vi "Dispense Function (SubVI).vi"(0 "Signals IN":T3={"Dispense"=FALSE, "Fill"=FALSE, "Spray"=FALSE, "Drain"=TRUE, "Complete"=FALSE, "Fill Error"=FALSE, "Dispense Error"=FALSE, "Fill Timeout"=FALSE, "Dispense Timeout"=FALSE}, 1 "Values IN":T4 {"Drain Time (s)" format="%.2f"; "Drain Rate (g/sec)" format="%.2f"; "Time Elapsed (s)" format="%.2f"; "Time Target (s)" format="%.2f"; "Dynamic Setpoint (g)" format="%.2f"; "Static Setpoint (g)" format="%.2f"; "Grams to Setpoint" format="%.2f"; "Adjusted Mass (g)" format="%.2f"; "Dispense Rate (g/sec)" format="%.2f"; "Fill Mass (g)" format="%.2f"; "Fill Rate (g/sec)" format="%.2f"}, 2 "Measured Mass (g)":dbl, 3 "Main Concentration Setpoint (%)":dbl, 4 "Product Weight (g)":dbl, 5 "Settings":T2={"ON Settings"={"Enable Dynamic Setpoint?"=TRUE, "Enable Dynamic Dispense Time?"=TRUE, "Enable Drain Rate Functions"=TRUE, "Dispense Sample Time (s)"=0.5, "Dispense Slope Ave"=0, "ON Timeout (sec)"=600.0, "1st Setpoint (% of Target)"=0.0, "2nd Setpoint (% of Target)"=0.0, "3rd Setpoint (% of Target)"=0.0, "Measure Dispense Delay (sec)"=0.0, "Settle Slope Sample Time (s)"=0.0}, "OFF Settings"={"Drain Sample Time (s)"=0.5, "Drain Rate Ave Size"=5, "Drain Rate Limits (± g/sec)"=10.0, "Level Slope Range (± g/sec)"=0.25, "OFF Timeout (sec)"=0.0, "Near SP Slope Level (± g/sec)"=0.01, "Near Setpoint Threshold (%)"=95.0}, "Overshoot Settings"={"Time Limit (s)"=60.0, "Container MAX (g)"=1500.0, "Max FILL Slope (+/- g/sec)"=10.0, "% Overshot to Enable (>)"=0.25}, "FILL Timeout (s)"=300.0, "Full Settle Time (s)"=20.0, "Pre-Hydrate \nSpray Time (s)"=10.0, "Pre-Hydrate \nWait Time (s)"=30.0}, 9 "Main Case Change?":bool) -> (14 "Signals OUT":T3={"Dispense"=FALSE, "Fill"=FALSE, "Spray"=FALSE, "Drain"=TRUE, "Complete"=FALSE, "Fill Error"=FALSE, "Dispense Error"=FALSE, "Fill Timeout"=FALSE, "Dispense Timeout"=FALSE}, 15 "Values OUT":T4 {"Drain Time (s)" format="%.2f"; "Drain Rate (g/sec)" format="%.2f"; "Time Elapsed (s)" format="%.2f"; "Time Target (s)" format="%.2f"; "Dynamic Setpoint (g)" format="%.2f"; "Static Setpoint (g)" format="%.2f"; "Grams to Setpoint" format="%.2f"; "Adjusted Mass (g)" format="%.2f"; "Dispense Rate (g/sec)" format="%.2f"; "Fill Mass (g)" format="%.2f"; "Fill Rate (g/sec)" format="%.2f"}, 16 "Spray Count":i32, 17 "Product Values":T1, 18 "Hydration (g)":dbl, 19 "Dispense Complete?":bool)   [LabVIEW 2009]
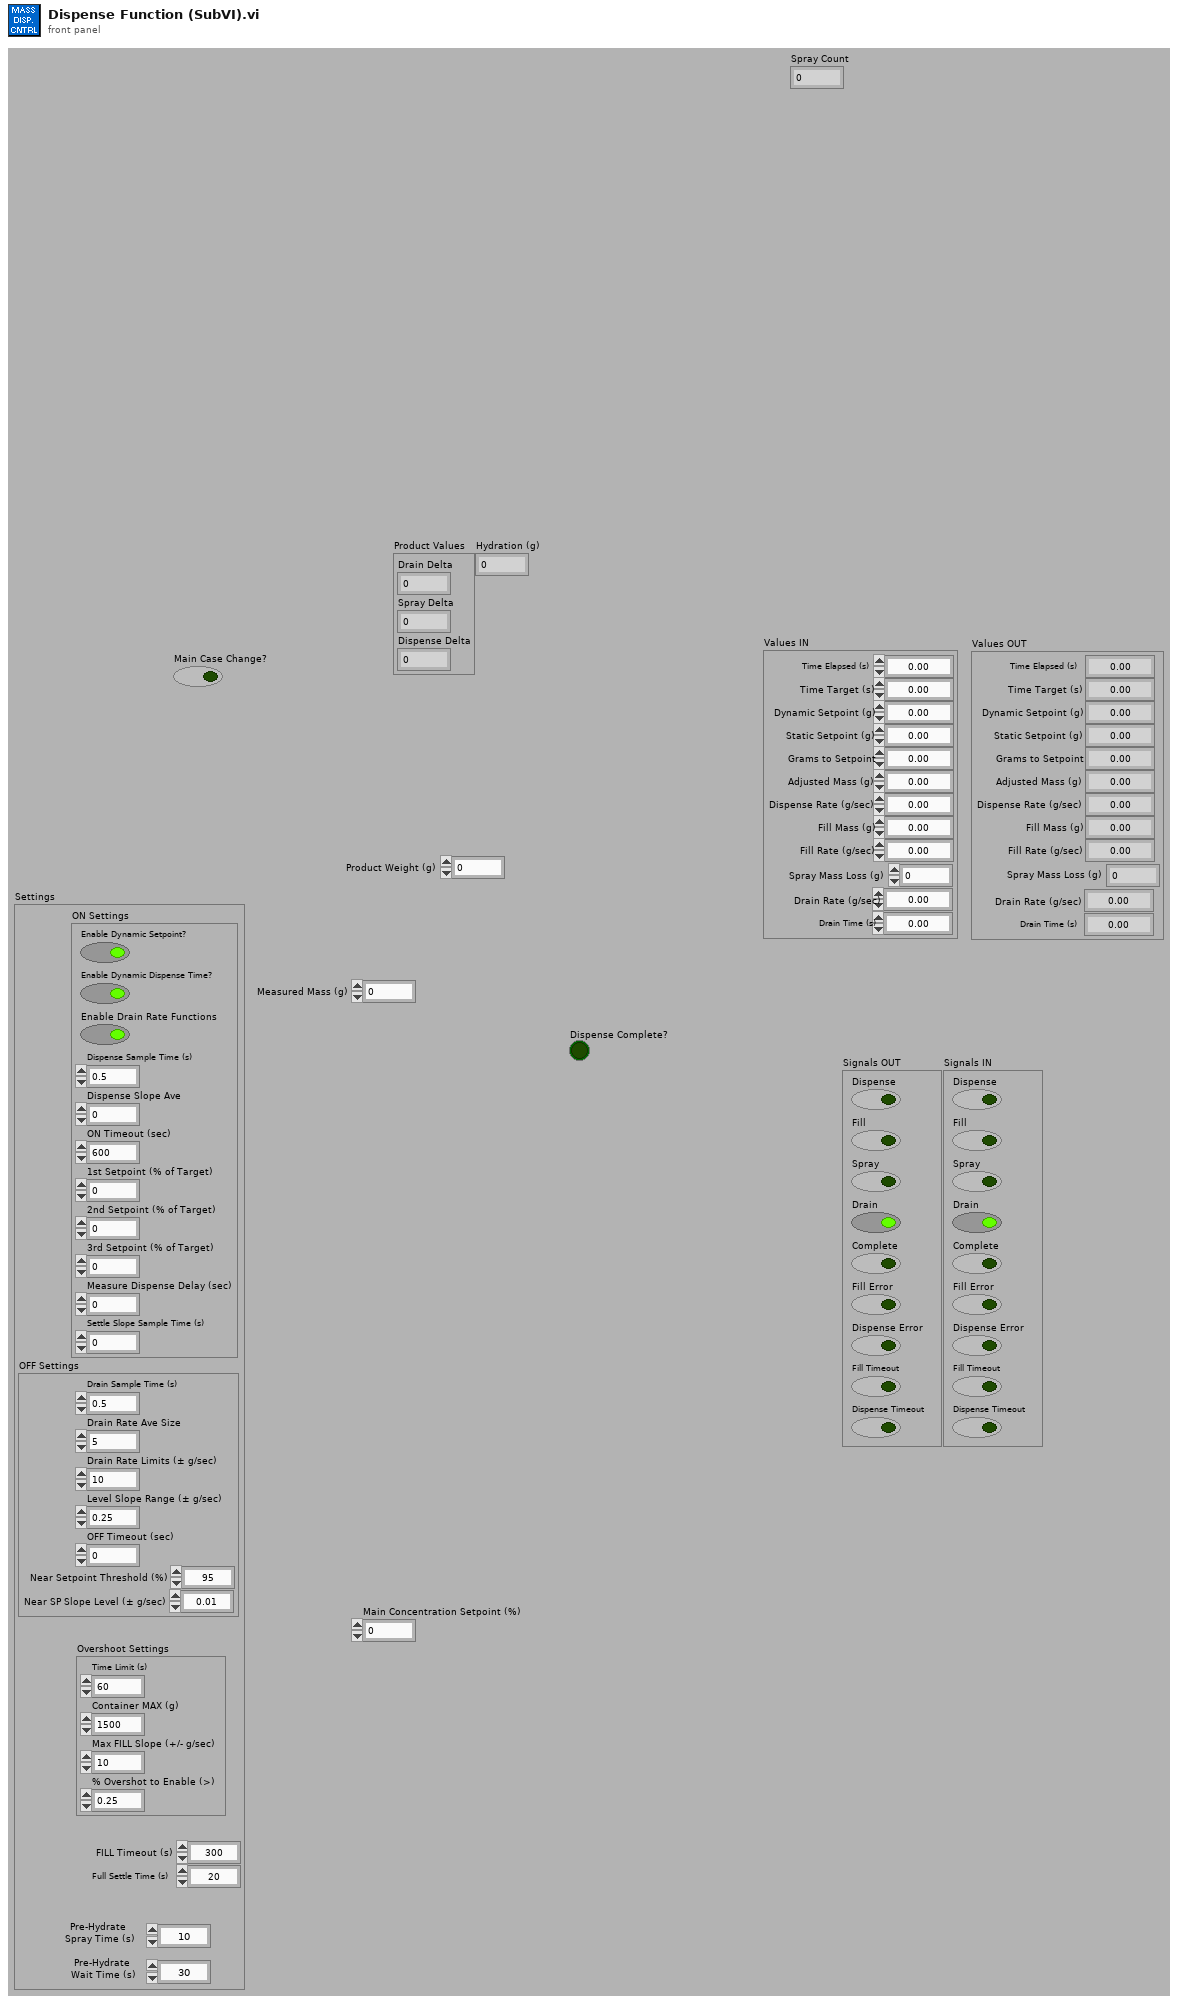
[diagram p1: front panel]
types:
  T1 = cluster{"Drain Delta":dbl, "Spray Delta":dbl, "Dispense Delta":dbl}
  T2 = cluster{"ON Settings":cluster{"Enable Dynamic Setpoint?":bool, "Enable Dynamic Dispense Time?":bool, "Enable Drain Rate Functions":bool, "Dispense Sample Time (s)":dbl, "Dispense Slope Ave":i32, "ON Timeout (sec)":dbl, "1st Setpoint (% of Target)":dbl, "2nd Setpoint (% of Target)":dbl, "3rd Setpoint (% of Target)":dbl, "Measure Dispense Delay (sec)":dbl, "Settle Slope Sample Time (s)":dbl}, "OFF Settings":cluster{"Drain Sample Time (s)":dbl, "Drain Rate Ave Size":i32, "Drain Rate Limits (± g/sec)":dbl, "Level Slope Range (± g/sec)":dbl, "OFF Timeout (sec)":dbl, "Near SP Slope Level (± g/sec)":dbl, "Near Setpoint Threshold (%)":dbl}, "Overshoot Settings":cluster{"Time Limit (s)":dbl, "Container MAX (g)":dbl, "Max FILL Slope (+/- g/sec)":dbl, "% Overshot to Enable (>)":dbl}, "FILL Timeout (s)":dbl, "Full Settle Time (s)":dbl, "Pre-Hydrate \nSpray Time (s)":dbl, "Pre-Hydrate \nWait Time (s)":dbl}
  T3 = cluster{"Dispense":bool, "Fill":bool, "Spray":bool, "Drain":bool, "Complete":bool, "Fill Error":bool, "Dispense Error":bool, "Fill Timeout":bool, "Dispense Timeout":bool}
  T4 = cluster{"Time Elapsed (s)":dbl, "Time Target (s)":dbl, "Dynamic Setpoint (g)":dbl, "Static Setpoint (g)":dbl, "Grams to Setpoint":dbl, "Adjusted Mass (g)":dbl, "Dispense Rate (g/sec)":dbl, "Fill Mass (g)":dbl, "Fill Rate (g/sec)":dbl, "Spray Mass Loss (g)":dbl, "Drain Rate (g/sec)":dbl, "Drain Time (s)":dbl}
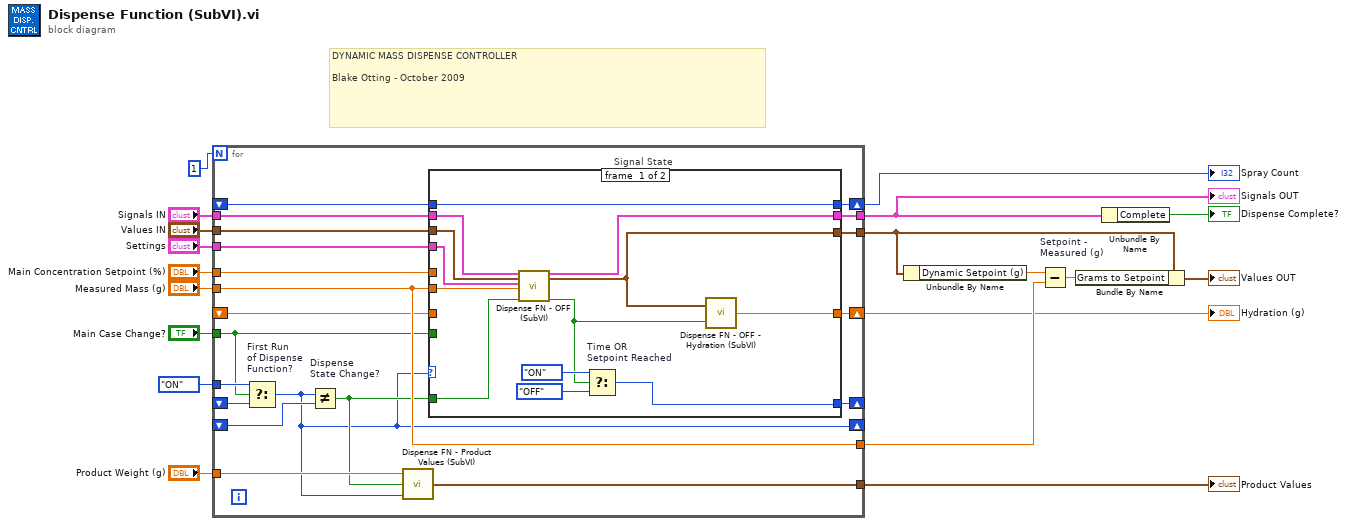
[diagram p0: block diagram]
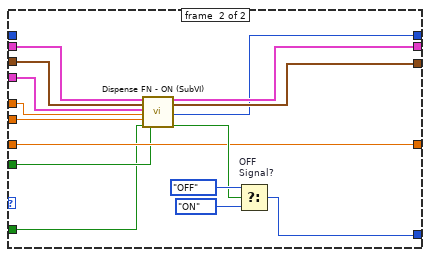
[diagram p2: hidden frame]
diagram:
  # "DYNAMIC MASS DISPENSE CONTROLLER\n\nBlake Otting - October 2009"
  n1 = for {
    N: 1 -> [_]
    tunnel: "Measured Mass (g)" -> [w33]
    tunnel: "Settings" -> [w39]
    shift-right: [w37] -> _
    shift-left: _ -> [w29]
    tunnel: "Main Concentration Setpoint (%)" -> [w38]
    tunnel: "Values IN" -> [w36]
    tunnel: [w35] -> w9
    tunnel: [w34] -> w12
    tunnel: "Signals IN" -> [w22]
    tunnel: [w33] -> w10
    shift-right: [w32] -> w6
    shift-left: _ -> [w31]
    tunnel: enum16{"OFF", "ON"}."ON" ("Signal State 2") -> [w30]
    tunnel: "Main Case Change?" -> [w24]
    tunnel: [w28] -> w3
    tunnel: "Product Weight (g)" -> [w27]
    shift-right: [w23] -> _
    shift-left: _ -> [w26]
    shift-right: [w21] -> w1
    shift-left: _ -> [w20]
    n2 = Select "First Run\nof Dispense\nFunction?"(t=w30, s=w24, f=w29) -> (s? t:f=w23:enum16{"OFF", "ON"})
    n3 = Not Equal? "Dispense\nState Change?"(x=w23, y=w26) -> (x != y?=w25:bool)
    n4 = call "Dispense FN - Product Values (SubVI).vi"("State Input"=w23, "Dispense State Change?"=w25, "Product Weight (g)"=w27) -> ("Product Values"=w28:T1)
    n5 = case "Signal State" shown="\"OFF\", Default" w23 {
      tunnel: w33 -> [w49 w57]
      tunnel: w39 -> [w41 w54]
      tunnel: [w51 w65] -> w37
      tunnel: w38 -> [_ w55]
      tunnel: w36 -> [w48 w60]
      tunnel: w22 -> [w47 w62]
      tunnel: [w45 w61] -> w35
      tunnel: [w46 w63] -> w34
      tunnel: [w43 w59] -> w32
      tunnel: w31 -> [_ w59]
      tunnel: w25 -> [w42 w56]
      tunnel: w24 -> [_ w58]
      tunnel: [w40 w53] -> w21
      tunnel: w20 -> [w40 _]
      frame #0 {
        n6 = call "Dispense FN - OFF (SubVI).vi"("Signals IN"=w47, "Values IN"=w48, "Settings"=w41, "Measured Mass (g)"=w49, "State Change?"=w42) -> ("Signals OUT"=w46:T3, "Values OUT"=w45:T4, "ON Signal"=w44:bool)  [unwired: 2 in, 10 out]
        n7 = Select "Time OR\nSetpoint Reached"(t=enum16{"OFF", "ON"}."ON" ("Mode (Read)"), s=w44, f=enum16{"OFF", "ON"}."OFF" ("Mode (Read)")) -> (s? t:f=w51:enum16{"OFF", "ON"})
        n8 = call "Dispense FN - OFF - Hydration (SubVI).vi"("ON Signal"=w44, "Values"=w45) -> ("Hydration (g)"=w43:dbl)
      }
      frame #1 {
        n9 = call "Dispense FN - ON (SubVI).vi"("Signals IN"=w62, "Values IN"=w60, "Settings"=w54, "Main Concentration Setpoint (%)"=w55, "Measured Mass (g)"=w57, "State Change?"=w56, "Main Case Change?"=w58) -> ("Signals OUT"=w63:T3, "Values OUT"=w61:T4, "Spray Count"=w53:i32, "OFF Signal"=w64:bool)  [unwired: 1 in, 8 out]
        n10 = Select "OFF\nSignal?"(t=enum16{"OFF", "ON"}."OFF" ("Signal State 2"), s=w64, f=enum16{"OFF", "ON"}."ON" ("Signal State 2")) -> (s? t:f=w65:enum16{"OFF", "ON"})
      }
    }
  }
  "Signals OUT" <- w12
  "Product Values" <- w3
  "Hydration (g)" <- w6
  "Spray Count" <- w1
  n11 = Unbundle By Name(w9) -> ("Dynamic Setpoint (g)"=w8:dbl)
  n12 = Subtract "Setpoint -\nMeasured (g)"(x=w8, y=w10) -> (x-y=w7:dbl)
  n13 = Bundle By Name(cluster=w9, "Grams to Setpoint"=w7) -> (→"Values OUT":T4)
  n14 = Unbundle By Name(w12) -> ("Complete"=→"Dispense Complete?":bool)
